vi "Loop Delay.vi"(11 "Loop Name":string) -> (3 "Timings":cluster{"Call Name":string, "Delta (ms)":u32}[](array[cluster]))   [LabVIEW 2013]
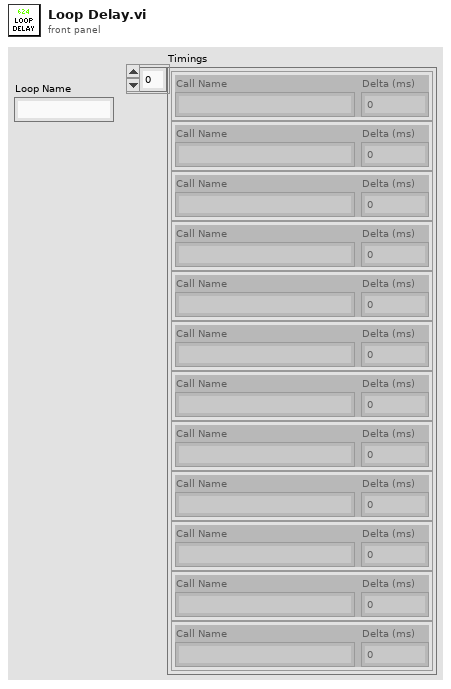
[diagram p1: front panel]
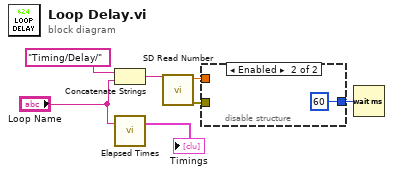
[diagram p0: block diagram]
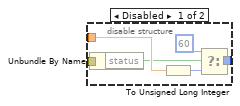
[diagram p2: hidden frame]
diagram:
  n1 = Concatenate Strings("Timing/Delay/" ("string"), "Loop Name") -> (w4:string)
  n2 = call "Elapsed Times.vi"("Call Name"="Loop Name") -> ("Timings"=→"Timings":cluster{"Call Name":string, "Delta (ms)":u32}[])  [unwired: 2 in]
  n3 = call <vilib>:"SD Read Number.vi"("Name"=w4) -> ("error out"=w6:errorcluster, "Numeric"=w7:dbl)  [unwired: 8 in, 1 out]
  n4 = disable-structure shown="Enabled" {
    disable-tunnel: w7 -> [w13 _]
    disable-tunnel: w6 -> [w12 _]
    disable-tunnel: [w10 u32 60 ("t")] -> w5
    frame Disabled {
      n5 = Unbundle By Name(w12) -> ("status"=w8:bool)
      n6 = To Unsigned Long Integer(number=w13) -> (unsigned 32bit integer=w11:u32)
      n7 = Select(t=u32 60, s=w8, f=w11) -> (s? t:f=w10:u32)
    }
    frame Enabled {
    }
  }
  n8 = Wait (ms)(milliseconds to wait=w5) -> ()  [unwired: 1 out]
